vi "Periodic Tasks.vi"(8 "error in":errorcluster) -> ()   [LabVIEW 2012]
doc: "This VI runs in parallel to other tasks. It can contain as many user-defined periodic loops as you need. These can carry out PID or other sorts of timed response."
uses:
  <vilib>/Rock Robotics/SystemInterfaces/Utilities/FPGA_UtilitiesLED Source.ctl
  <vilib>/Rock Robotics/SystemInterfaces/Utilities/FPGA_UtilitiesLED State.ctl
  Robot Global Data.vi
  <vilib>/Rock Robotics/WPI/Ultrasonic/WPI_UltrasonicRangeUnits.ctl
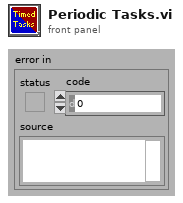
[diagram p1: front panel]
types:
  T1 = typedef "FPGA_UtilitiesLED State.ctl" = enum16{"Off", "On", "Toggle"}
  T2 = typedef "FPGA_UtilitiesLED Source.ctl" = enum16{"User LED", "FPGA LED"}
  T3 = typedef "WPI_UltrasonicRangeUnits.ctl" = enum16{"inches", "mm"}
  T4 = typedef "WPI_UltrasonicDeviceRef.ctl" = cluster{"DevStatus":errorcluster, "Ping Digital Module":T5, "Echo Digital Module":T5, "Ping Channel":T6, "Echo Channel":T6, "CntIndex":T7}
  T5 = typedef "FPGA_TypedefDigitalModule.ctl" = enum16{"Digital Module 1", "Digital Module 2"}
  T6 = typedef "FPGA_DIOChannel.ctl" = enum8{"DIO 1", "DIO 2", "DIO 3", "DIO 4", "DIO 5", "DIO 6", "DIO 7", "DIO 8", "DIO 9", "DIO 10", "DIO 11", "DIO 12", "DIO 13", "DIO 14", "Invalid"}
  T7 = typedef "FPGA_CounterCtrSystemIndex.ctl" = enum8{"Ctr 0", "Ctr 1", "Ctr 2", "Ctr 3", "Ctr 4", "Ctr 5", "Ctr 6", "Ctr 7", "Invalid"}
  T8 = typedef "WPI_DigitalOutputDevRef.ctl" = cluster{"Digital Module":T5, "DIO Channel":T6, "DevStatus":errorcluster}
  T9 = typedef "WPI_CounterDevRef.ctl" = cluster{"DevStatus":errorcluster, "CntIndex":T7}
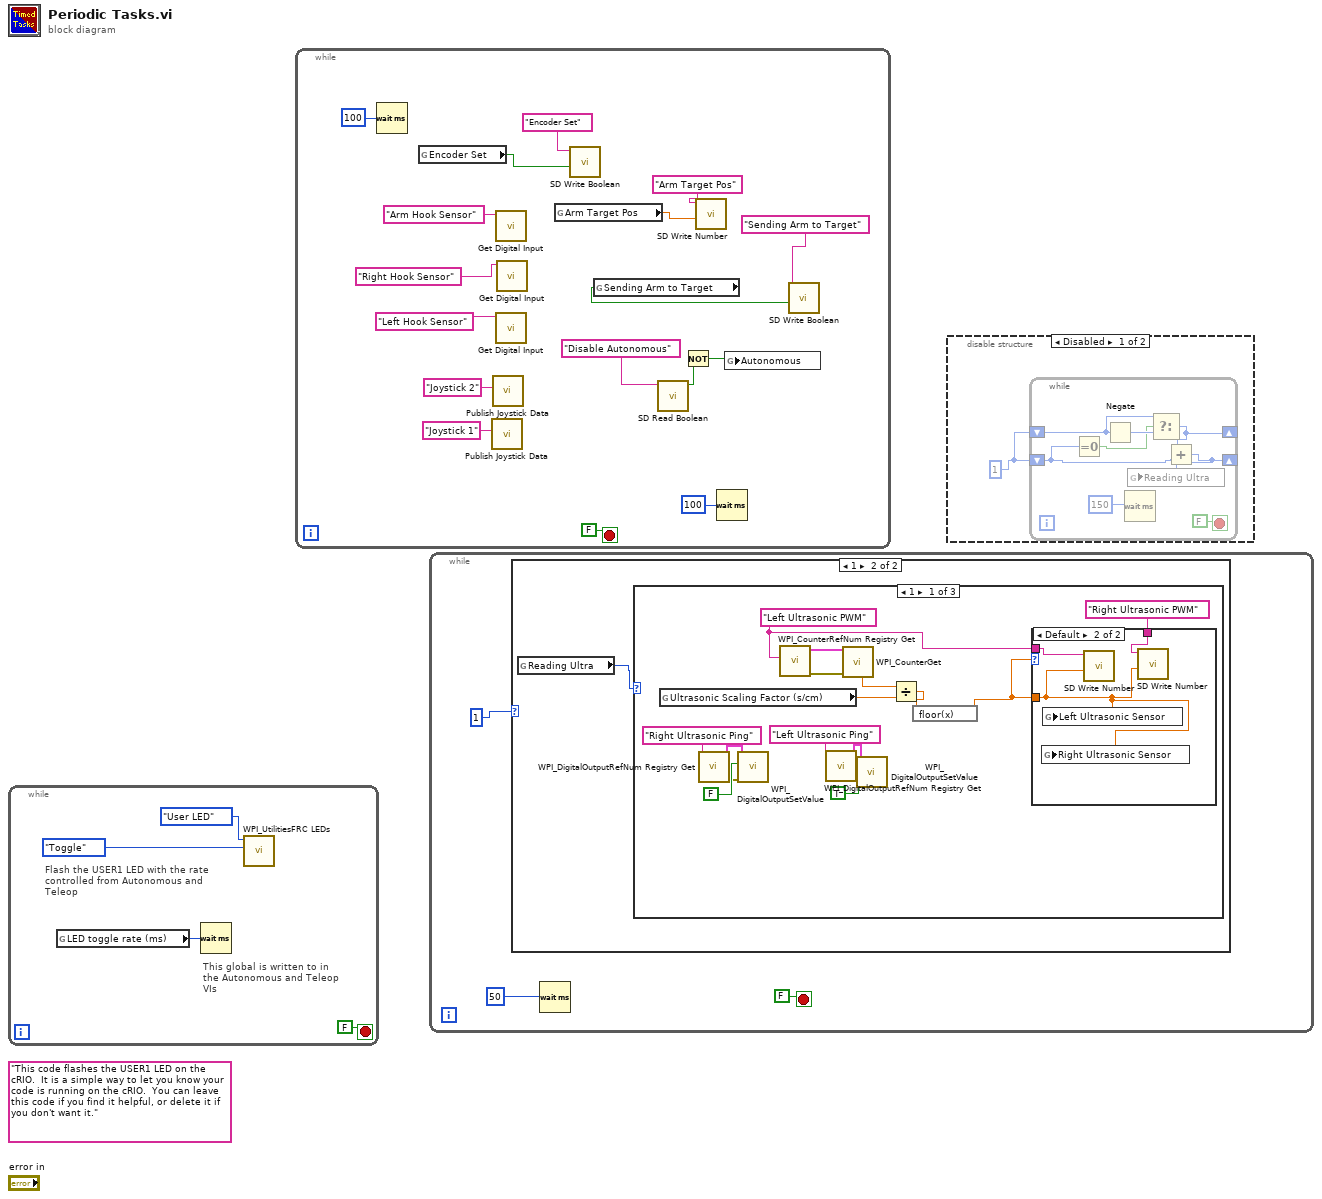
[diagram p0: block diagram]
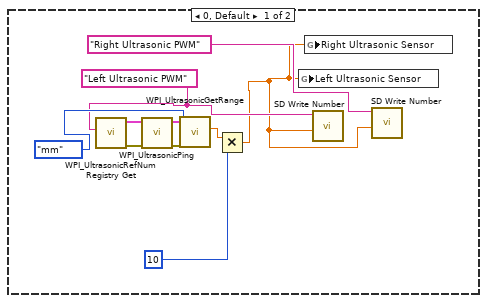
[diagram p3: hidden frame]
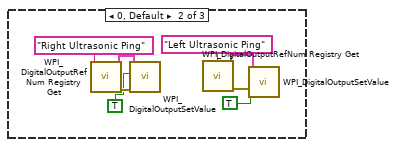
[diagram p5: hidden frame]
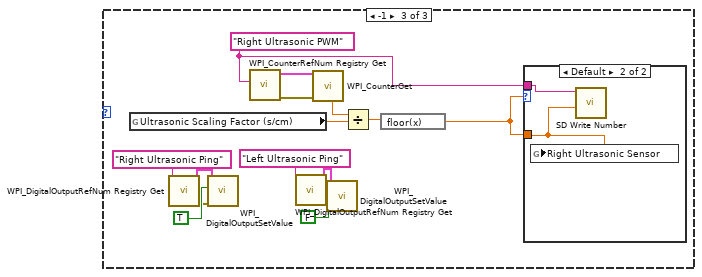
[diagram p6: hidden frame]
diagram:
  (unwired) "This code flashes the USER1 LED on the cRIO.  It is a simple way to let you know your code is running on the cRIO.  You can leave this code if you find it helpful, or delete it if you don't want it."
  n1 = while {
    stop <- FALSE stop-if-true
    # "This global is written to in the Autonomous and Teleop VIs"
    # "Flash the USER1 LED with the rate controlled from Autonomous and Teleop"
    n2 = global read "Robot Global Data.vi" "LED toggle rate (ms)"() -> (w1:u32)
    n3 = Wait (ms)(milliseconds to wait=w1) -> ()  [unwired: 1 out]
    n4 = call <vilib>:"WPI_UtilitiesFRC LEDs.vi"("State"=FPGA_UtilitiesLED_State."Toggle", "LED Type"=FPGA_UtilitiesLED_Source."User LED") -> ()  [unwired: 1 in, 9 out]
  }
  n5 = while {
    stop <- FALSE stop-if-true
    n6 = Wait (ms)(milliseconds to wait=u32 100) -> ()  [unwired: 1 out]
    n7 = global read "Robot Global Data.vi" "Encoder Set"() -> (w13:bool)
    n8 = call "Publish Joystick Data.vi"("Joystick Refnum"="Joystick 1") -> ()  [unwired: 11 in]
    n9 = call "Publish Joystick Data.vi"("Joystick Refnum"="Joystick 2") -> ()  [unwired: 11 in]
    n10 = call "Get Digital Input.vi"("DigitalInput Refnum"="Arm Hook Sensor") -> ()  [unwired: 10 in, 1 out]
    n11 = call "Get Digital Input.vi"("DigitalInput Refnum"="Left Hook Sensor") -> ()  [unwired: 10 in, 1 out]
    n12 = call "Get Digital Input.vi"("DigitalInput Refnum"="Right Hook Sensor") -> ()  [unwired: 10 in, 1 out]
    n13 = global read "Robot Global Data.vi" "Arm Target Pos"() -> (w9:dbl)
    n14 = call <vilib>:"SD Write Boolean.vi"("Boolean"=w13, "Name"="Encoder Set") -> ()  [unwired: 8 in, 2 out]
    n15 = global read "Robot Global Data.vi" "Sending Arm to Target"() -> (w10:bool)
    n16 = call <vilib>:"SD Read Boolean.vi"("Name"="Disable Autonomous") -> ("Boolean"=w6:bool)  [unwired: 8 in, 2 out]
    n17 = Not(x=w6) -> (.not. x?=w7:bool)
    n18 = call <vilib>:"SD Write Number.vi"("Numeric"=w9, "Name"="Arm Target Pos") -> ()  [unwired: 8 in, 2 out]
    n19 = Wait (ms)(milliseconds to wait=u32 100) -> ()  [unwired: 1 out]
    n20 = global write "Robot Global Data.vi" "Autonomous"(w7) -> ()
    n21 = call <vilib>:"SD Write Boolean.vi"("Boolean"=w10, "Name"="Sending Arm to Target") -> ()  [unwired: 8 in, 2 out]
  }
  n22 = while {
    stop <- FALSE stop-if-true
    n23 = case shown="1" 1 {
      frame 0, Default {
        w29 = "Left Ultrasonic PWM"
        n24 = call <vilib>:"WPI_UltrasonicRefNum Registry Get.vi"("refnum name"=w29) -> ("error out"=w32:errorcluster, "UltrasonicDevRef"=w31:T4)  [unwired: 9 in]
        n25 = call <vilib>:"WPI_UltrasonicPing.vi"("error in (no error)"=w32, "UltrasonicDevRef"=w31) -> ("error out"=w34:errorcluster, "UltrasonicDevRef"=w33:T4)  [unwired: 8 in]
        n26 = call <vilib>:"WPI_UltrasonicGetRange.vi"("error in (no error)"=w34, "Range Units"=WPI_UltrasonicRangeUnits."mm", "UltrasonicDevRef"=w33) -> ("Distance"=w27:dbl)  [unwired: 6 in, 2 out]
        n27 = Multiply(x=w27, y=10) -> (x*y=w25:dbl)
        n28 = global write "Robot Global Data.vi" "Left Ultrasonic Sensor"(w25) -> ()
        n29 = global write "Robot Global Data.vi" "Right Ultrasonic Sensor"(w25) -> ()
        n30 = call <vilib>:"SD Write Number.vi"("Numeric"=w25, "Name"=w29) -> ()  [unwired: 8 in, 2 out]
        n31 = call <vilib>:"SD Write Number.vi"("Numeric"=w25, "Name"="Right Ultrasonic PWM") -> ()  [unwired: 8 in, 2 out]
      }
      frame 1 {
        n32 = global read "Robot Global Data.vi" "Reading Ultra"() -> (w35:i32)
        n33 = case shown="1" w35 {
          frame 1 {
            w39 = "Left Ultrasonic PWM"
            n34 = global read "Robot Global Data.vi" "Ultrasonic Scaling Factor (s/cm)"() -> (w48:dbl)
            n35 = call <vilib>:"WPI_DigitalOutputRefNum Registry Get.vi"("refnum name"="Right Ultrasonic Ping") -> ("error out"=w41:errorcluster, "DigitalOutputDevRef"=w42:T8)  [unwired: 9 in]
            n36 = call <vilib>:"WPI_DigitalOutputSetValue.vi"("error in (no error)"=w41, "Value"=FALSE, "DigitalOutputDevRef"=w42) -> ()  [unwired: 7 in, 2 out]
            n37 = call <vilib>:"WPI_CounterRefNum Registry Get.vi"("refnum name"=w39) -> ("error out"=w50:errorcluster, "CounterDevRef"=w51:T9)  [unwired: 9 in]
            n38 = call <vilib>:"WPI_DigitalOutputRefNum Registry Get.vi"("refnum name"="Left Ultrasonic Ping") -> ("error out"=w46:errorcluster, "DigitalOutputDevRef"=w45:T8)  [unwired: 9 in]
            n39 = call <vilib>:"WPI_CounterGet.vi"("error in (no error)"=w50, "CounterDevRef in"=w51) -> ("Period (sec)"=w49:dbl)  [unwired: 4 in, 5 out]
            n40 = call <vilib>:"WPI_DigitalOutputSetValue.vi"("error in (no error)"=w46, "Value"=TRUE, "DigitalOutputDevRef"=w45) -> ()  [unwired: 7 in, 2 out]
            n41 = Divide(x=w49, y=w48) -> (x/y=w38:dbl)
            n42 = expression code="floor(x)"(w38) -> (w37:dbl)
            n43 = case shown="Default" w37 {
              tunnel: w37 -> [_ w53]
              tunnel: w39 -> [_ w54]
              tunnel: "Right Ultrasonic PWM" -> [_ w52]
              frame 0 {
              }
              frame Default {
                n44 = global write "Robot Global Data.vi" "Right Ultrasonic Sensor"(w53) -> ()
                n45 = global write "Robot Global Data.vi" "Left Ultrasonic Sensor"(w53) -> ()
                n46 = call <vilib>:"SD Write Number.vi"("Numeric"=w53, "Name"=w54) -> ()  [unwired: 8 in, 2 out]
                n47 = call <vilib>:"SD Write Number.vi"("Numeric"=w53, "Name"=w52) -> ()  [unwired: 8 in, 2 out]
              }
            }
          }
          frame 0, Default {
            n48 = call <vilib>:"WPI_DigitalOutputRefNum Registry Get.vi"("refnum name"="Right Ultrasonic Ping") -> ("error out"=w57:errorcluster, "DigitalOutputDevRef"=w58:T8)  [unwired: 9 in]
            n49 = call <vilib>:"WPI_DigitalOutputSetValue.vi"("error in (no error)"=w57, "Value"=TRUE, "DigitalOutputDevRef"=w58) -> ()  [unwired: 7 in, 2 out]
            n50 = call <vilib>:"WPI_DigitalOutputRefNum Registry Get.vi"("refnum name"="Left Ultrasonic Ping") -> ("error out"=w61:errorcluster, "DigitalOutputDevRef"=w60:T8)  [unwired: 9 in]
            n51 = call <vilib>:"WPI_DigitalOutputSetValue.vi"("error in (no error)"=w61, "Value"=TRUE, "DigitalOutputDevRef"=w60) -> ()  [unwired: 7 in, 2 out]
          }
          frame -1 {
            w65 = "Right Ultrasonic PWM"
            n52 = global read "Robot Global Data.vi" "Ultrasonic Scaling Factor (s/cm)"() -> (w74:dbl)
            n53 = call <vilib>:"WPI_DigitalOutputRefNum Registry Get.vi"("refnum name"="Right Ultrasonic Ping") -> ("error out"=w67:errorcluster, "DigitalOutputDevRef"=w68:T8)  [unwired: 9 in]
            n54 = call <vilib>:"WPI_DigitalOutputSetValue.vi"("error in (no error)"=w67, "Value"=TRUE, "DigitalOutputDevRef"=w68) -> ()  [unwired: 7 in, 2 out]
            n55 = call <vilib>:"WPI_CounterRefNum Registry Get.vi"("refnum name"=w65) -> ("error out"=w76:errorcluster, "CounterDevRef"=w77:T9)  [unwired: 9 in]
            n56 = call <vilib>:"WPI_DigitalOutputRefNum Registry Get.vi"("refnum name"="Left Ultrasonic Ping") -> ("error out"=w72:errorcluster, "DigitalOutputDevRef"=w71:T8)  [unwired: 9 in]
            n57 = call <vilib>:"WPI_CounterGet.vi"("error in (no error)"=w76, "CounterDevRef in"=w77) -> ("Period (sec)"=w75:dbl)  [unwired: 4 in, 5 out]
            n58 = call <vilib>:"WPI_DigitalOutputSetValue.vi"("error in (no error)"=w72, "Value"=FALSE, "DigitalOutputDevRef"=w71) -> ()  [unwired: 7 in, 2 out]
            n59 = Divide(x=w75, y=w74) -> (x/y=w64:dbl)
            n60 = expression code="floor(x)"(w64) -> (w63:dbl)
            n61 = case shown="Default" w63 {
              tunnel: w63 -> [_ w79]
              tunnel: w65 -> [_ w78]
              frame 0 {
              }
              frame Default {
                n62 = global write "Robot Global Data.vi" "Right Ultrasonic Sensor"(w79) -> ()
                n63 = call <vilib>:"SD Write Number.vi"("Numeric"=w79, "Name"=w78) -> ()  [unwired: 8 in, 2 out]
              }
            }
          }
        }
      }
    }
    n64 = Wait (ms)(milliseconds to wait=u32 50) -> ()  [unwired: 1 out]
  }
  n65 = disable-structure shown="Disabled" {
    frame Disabled {
      w80 = 1
      n66 = while {
        shift-right: [w81] -> _
        shift-left: w80 -> [w82]
        shift-right: [w83] -> _
        shift-left: w80 -> [w85]
        stop <- FALSE stop-if-true
        n67 = Equal To 0?(x=w82) -> (x = 0?=w84:bool)
        n68 = Negate(x=w85) -> (-x=w86:i32)
        n69 = Wait (ms)(milliseconds to wait=150) -> ()  [unwired: 1 out]
        n70 = Select(t=w85, s=w84, f=w86) -> (s? t:f=w83:i32)
        n71 = Add(x=w83, y=w82) -> (x+y=w81:i32)
        n72 = global write "Robot Global Data.vi" "Reading Ultra"(w81) -> ()
      }
    }
    frame Enabled {
    }
  }
